vi "Logic_Export_Raw_Digital_to_CSV.vi"(4 "error in (no error)":errorcluster, 5 "Enabled Digital Channels":i32[](array[numeric]), 6 "Filepath Input":string, 7 "Session Ref In":T1) -> (0 "error out":errorcluster, 3 "Session Ref Out":T1)   [LabVIEW 2023]
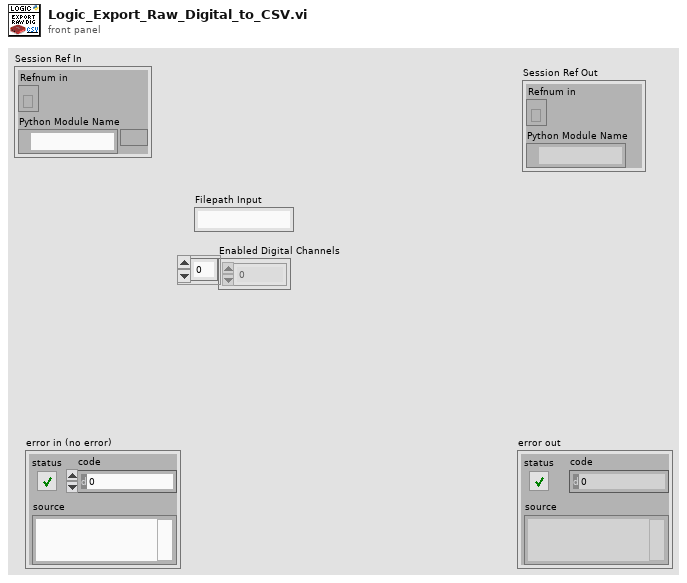
[diagram p1: front panel]
types:
  T1 = cluster{"Refnum in":refnum<k35>, "Python Module Name":path}
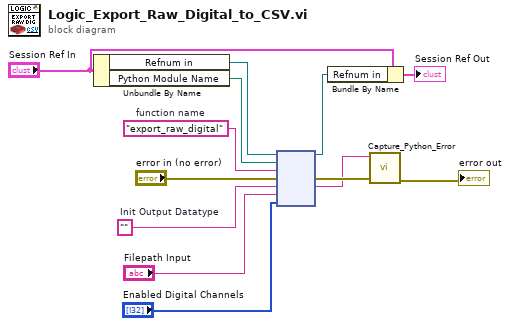
[diagram p0: block diagram]
diagram:
  w12 = "export_raw_digital"  # function name
  w11 = ""  # Init Output Datatype
  n1 = Unbundle By Name("Session Ref In") -> ("Refnum in"=w10:refnum<k35>, "Python Module Name"=w9:path)
  n2 = node(w10, w9, w12, "error in (no error)", w11, "Filepath Input", "Enabled Digital Channels") -> (w7:refnum<k35>, w3:errorcluster, w1:string)  [unwired: 2 in, 2 out]
  n3 = Bundle By Name(cluster="Session Ref In", "Refnum in"=w7) -> (→"Session Ref Out":T1)
  n4 = call "Capture_Python_Error.vi"("error in (no error)"=w3, "Error Message (start with ERROR)"=w1) -> ("error out"=→"error out":errorcluster)  [unwired: 9 in]
